vi "AddDebugInfoPathAndDepth.vi"(7 "Message":string, 8 "error in (no error)":errorcluster, 9 "Path":path, 11 "CDebugInfo in":refnum<class "CDebugInfo.lvclass">) -> (0 "error out":errorcluster, 3 "CDebugInfo out":refnum<class "CDebugInfo.lvclass">)   [LabVIEW 2020, in "DependencyInspection.lvlib" / "CDebugInfo.lvclass"]
uses:
  CDebugInfo.lvclass
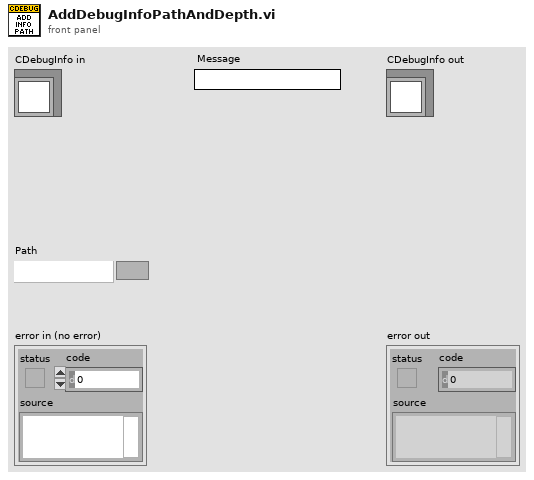
[diagram p1: front panel]
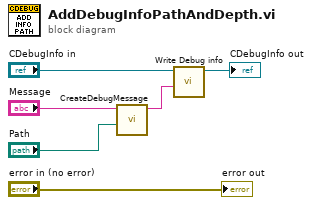
[diagram p0: block diagram]
diagram:
  n1 = call "CreateDebugMessage.vi"("Path"="Path", "Message"="Message") -> ("Debug message"=w3:string)  [unwired: 9 in]
  n2 = call-dynamic "Write Debug info.vi"("Debug info"=w3, "CDebugInfo in"="CDebugInfo in") -> ("CDebugInfo out"=→"CDebugInfo out":refnum<class "CDebugInfo.lvclass">)  [unwired: 9 in]
  "error out" <- "error in (no error)"
